vi "Sub Initialize.vi"(6 "Controller name":string, 8 "error in (no error)":errorcluster, 11 "Spectrum Recorder in":refnum<class "Spectrum Recorder.lvclass">) -> (0 "error out":errorcluster, 2 "Initialize Result":refnum<class "Acquired Result.lvclass">, 3 "Spectrum Recorder out":refnum<class "Spectrum Recorder.lvclass">)   [LabVIEW 2024, in "Spectrum Recorder.lvclass"]
uses:
  Spectrum Recorder.lvclass
  Spectrum Recorder.lvclass/Spectrum Recorder.ctl
  NHMFL_Core/Libraries/Red Pitaya/RP Core/RP Transceiver/Receiver format.ctl
  NHMFL_Core/Libraries/Red Pitaya/RP Core/RP Transceiver/RP Transceiver.lvclass
  NHMFL_Core/Libraries/Instruments/Instrument Driver/Worker State.ctl
  NHMFL_Core/Libraries/Instruments/Results/Acquired Result/Acquired Result.lvclass
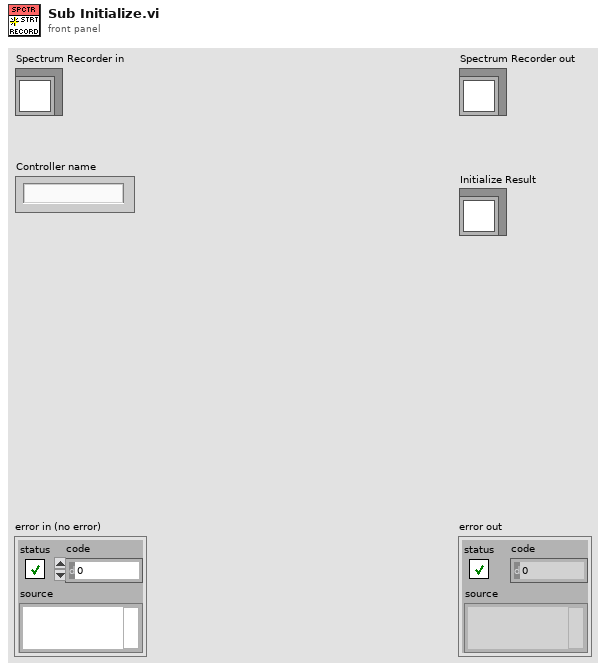
[diagram p1: front panel]
types:
  T1 = typedef "Receiver format.ctl" = enum16{"X-Y-F", "F-X-Y", "X-Y", "X"}
  T2 = typedef "Worker State.ctl" = enum16{"Idle", "Starting", "Working", "Stopping"}
  T3 = typedef "Spectrum Recorder Configuration.ctl" = cluster{"Start":dbl, "End":dbl, "Duration":dbl, "Filter time constant":dbl, "Repeat (-1: forever)":i32, "Update rate":dbl, "Data storage folder":path}
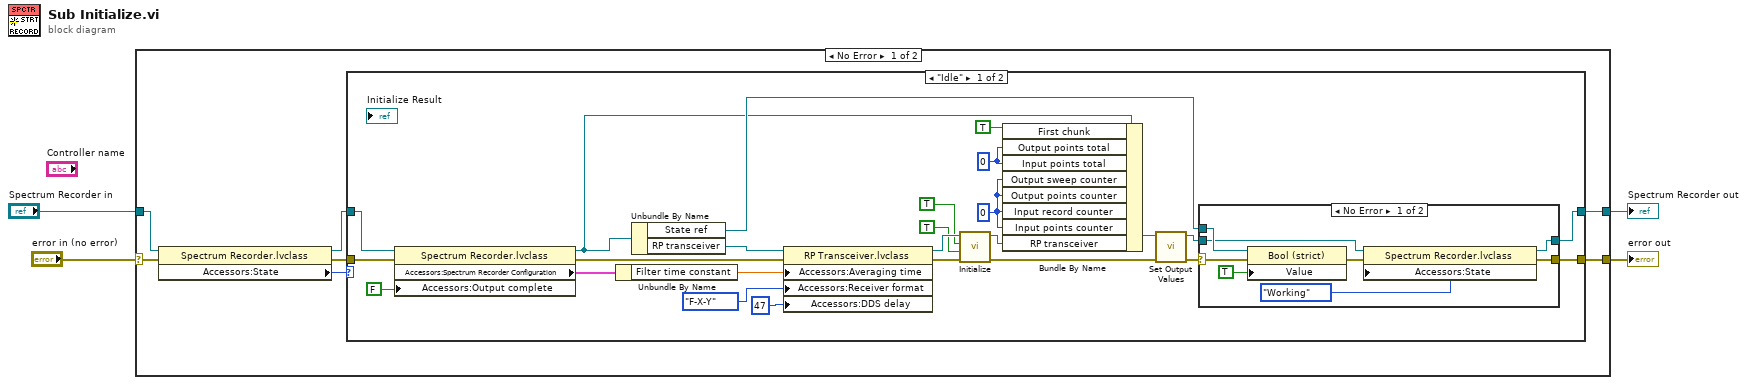
[diagram p0: block diagram]
diagram:
  n1 = case shown="No Error" "error in (no error)" {
    selector: "error in (no error)" -> [w6 w50]
    tunnel: [w9 w50] -> w3
    tunnel: [w11 w49] -> w1
    tunnel: "Spectrum Recorder in" -> [w10 w49]
    frame No Error {
      n2 = property class="Spectrum Recorder.lvclass"(reference=w10, error in=w6) -> (reference out=w8:refnum<class "Spectrum Recorder.lvclass">, error out=w5:errorcluster, "Accessors:State"=w7:T2)
      n3 = case shown="\"Idle\"" w7 {
        tunnel: w8 -> [w18 w48]
        tunnel: [w20 w48] -> w11
        tunnel: w5 -> [w14 w47]
        tunnel: [w27 w47] -> w9
        frame "Idle" {
          w19 = i64 0 ("Output points total")
          w25 = 0 ("Output sweep counter")
          n4 = property class="Spectrum Recorder.lvclass"(reference=w18, error in=w14, "Accessors:Output complete"=FALSE ("Output complete")) -> (reference out=w17:refnum<class "Spectrum Recorder.lvclass">, error out=w13:errorcluster, "Accessors:Spectrum Recorder Configuration"=w16:T3)
          n5 = Unbundle By Name(w16) -> ("Filter time constant"=w15:dbl)
          n6 = Unbundle By Name(w17) -> ("State ref"=w26:refnum<vi>, "RP transceiver"=w29:refnum<class "RP Transceiver.lvclass">)
          n7 = property class="RP Transceiver.lvclass"(reference=w29, error in=w13, "Accessors:Averaging time"=w15, "Accessors:Receiver format"=Receiver_format."F-X-Y" ("Receiver format"), "Accessors:DDS delay"=u32 47 ("DDS delay")) -> (reference out=w34:refnum<class "RP Transceiver.lvclass">, error out=w33:errorcluster)
          n8 = call-dynamic "Initialize.vi"("error in (no error)"=w33, "Send \"Connect client\""=TRUE ("Send \"Connect client\""), "Reset"=TRUE, "RP Transceiver in"=w34) -> ("error out"=w30:errorcluster, "RP Transceiver out"=w23:refnum<class "RP Transceiver.lvclass">)  [unwired: 6 in]
          n9 = Bundle By Name(cluster=w17, "First chunk"=TRUE, "Output points total"=w19, "Input points total"=w19, "Output sweep counter"=w25, "Output points counter"=w25, "Input record counter"=w25, "Input points counter"=w25, "RP transceiver"=w23) -> (w28:refnum<class "Spectrum Recorder.lvclass">)
          n10 = call-dynamic "Set Output Values.vi"("error in (no error)"=w30, "Spectrum Recorder in"=w28) -> ("error out"=w22:errorcluster, "Spectrum Recorder out"=w21:refnum<class "Spectrum Recorder.lvclass">)  [unwired: 8 in]
          n11 = case shown="No Error" w22 {
            selector: w22 -> [w43 w45]
            tunnel: [w38 w45] -> w27
            tunnel: w26 -> [w44 _]
            tunnel: w21 -> [w42 w46]
            tunnel: [w41 w46] -> w20
            frame No Error {
              n12 = property class="Bool (strict)"(reference=w44, error in=w43, "Value"=TRUE) -> (error out=w39:errorcluster)  [unwired: 1 out]
              n13 = property class="Spectrum Recorder.lvclass"(reference=w42, error in=w39, "Accessors:State"=Worker_State."Working" ("State")) -> (reference out=w41:refnum<class "Spectrum Recorder.lvclass">, error out=w38:errorcluster)
            }
            frame Error {
            }
          }
        }
        frame "Starting", Default {
        }
      }
    }
    frame Error {
    }
  }
  "error out" <- w3
  "Spectrum Recorder out" <- w1
